vi "loopTimer_us.vi"(1 "loop time set (us)":u32=100) -> (0 "loop time actual (us)":u32)   [LabVIEW 2016]
panel:
  # "This VI returns the time difference between sucessive calls.\nUsing a feedback node without a loop was made possible in LabVIEW 8.5.  This node will always return 0 on its first call."
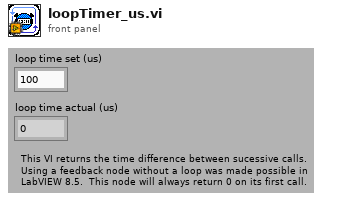
[diagram p1: front panel]
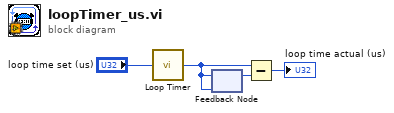
[diagram p0: block diagram]
diagram:
  n1 = call "Loop Timer"("Count(uSec)"="loop time set (us)") -> ("Tick Count(uSec)"=w2:u32)
  n2 = feedback-in #1(w2) -> ()
  n3 = feedback #1(w2) -> (w3:u32)
  n4 = Subtract(x=w2, y=w3) -> (x-y=→"loop time actual (us)":u32)
